vi "Configure.vi"(8 "error in (no error)":errorcluster, 11 "AOTF in":refnum<class "AOTF.lvclass">) -> (0 "error out":errorcluster, 2 "cancelled?":bool, 3 "AOTF out":refnum<class "AOTF.lvclass">)   [LabVIEW 2012, in "AOTF.lvclass"]
doc: "The configure method configures the details for the RabbitMQ connection. \n\nIn the derived class, make a call to the parent for setting these parameters."
uses:
  AOTF.lvclass
  <vilib>/Utility/miscctls.llb/LVPointTypeDef.ctl
  AOTF.lvclass/AOTF.ctl
  <vilib>/Distrio/Murmex/Murmex/Murmex.lvclass
  Controls/LUT path cluster.ctl
panel:
  in  "Tab Control":enum32{"Comport", "Debug"}(tab)
  in  "DO lines":tag
  in  "AO channel":tag
  in  "LUT561":path=path "D:/CLSM_Project/AOTF/561nm.txt" caption="LUT 561nm"
  in  "LUT515":path=path "D:/CLSM_Project/AOTF/515nm.txt" caption="LUT 515nm"
  in  "LUT491":path=path "D:/CLSM_Project/AOTF/491nm.txt" caption="LUT 491nm"
  in  "LUT445":path=path "D:/CLSM_Project/AOTF/445nm.txt" caption="LUT 445nm"
  in  "LUT405":path=path "D:/CLSM_Project/AOTF/405nm.txt" caption="LUT 405nm"
  in  "button::configure murmex":bool
  in  "button::ok":bool
  in  "button::cancel":bool
  # "RabbitMQ parameters"
  # "Window position"
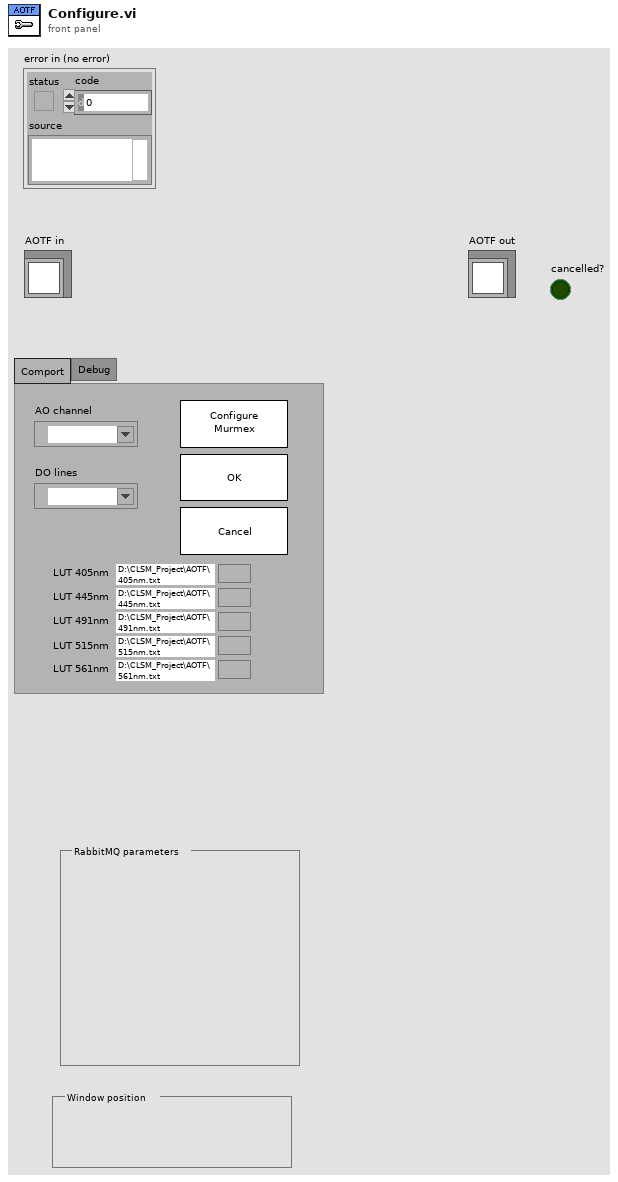
[diagram p1: front panel]
types:
  T1 = typedef "LVPointTypeDef.ctl" = cluster{"Horizontal":i16, "Vertical":i16}
  T2 = typedef "LUT path cluster.ctl" = cluster{"LUT path Array":path[]}
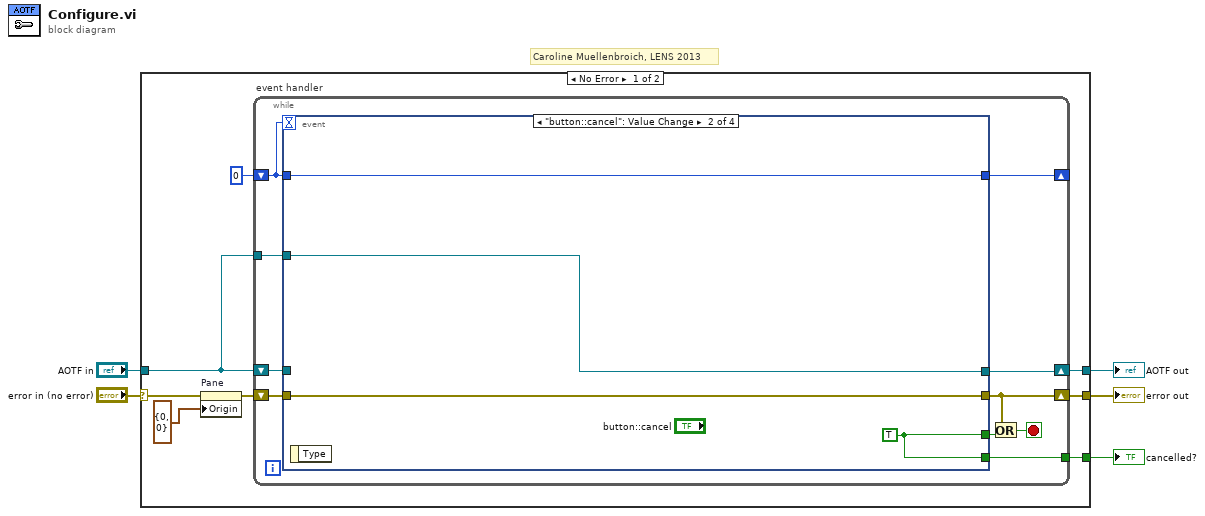
[diagram p0: block diagram]
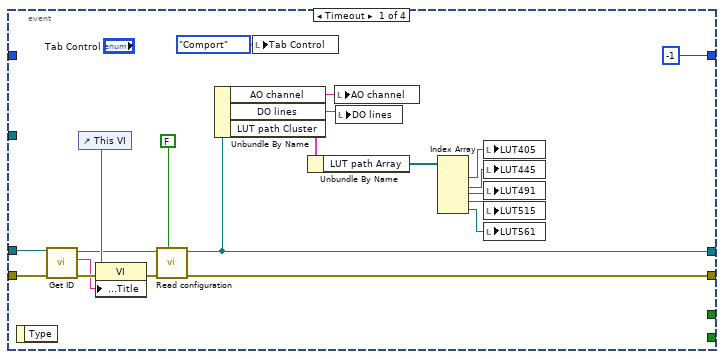
[diagram p2: hidden frame]
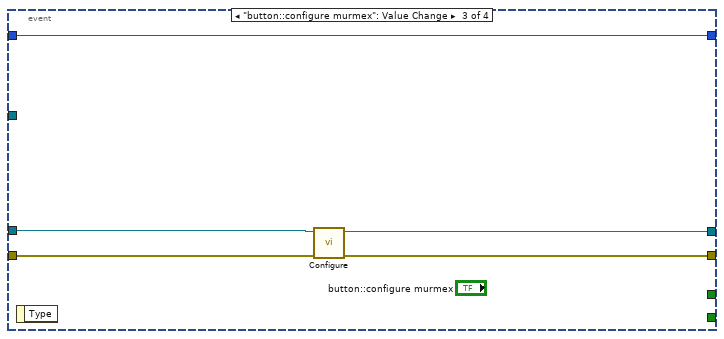
[diagram p3: hidden frame]
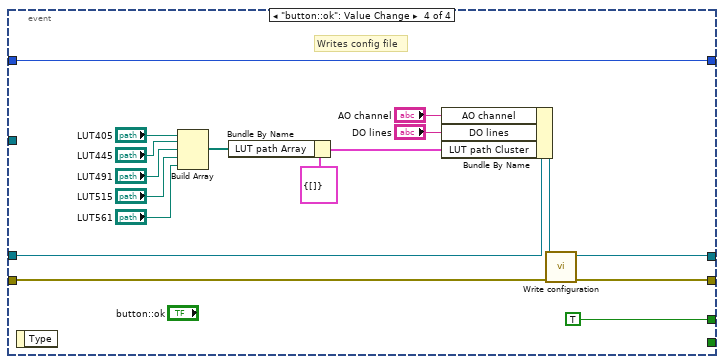
[diagram p4: hidden frame]
diagram:
  # "Caroline Muellenbroich, LENS 2013"
  n1 = case shown="No Error" "error in (no error)" {
    selector: "error in (no error)" -> [w11 w71]
    tunnel: "AOTF in" -> [w12 w72]
    tunnel: [w8 w71] -> w1
    tunnel: [w7 w72] -> w3
    tunnel: [w6 _] -> w2
    frame No Error {
      n2 = property on="Pane" class="Pane"(error in=w11, "Origin"=T1 {"Horizontal"=0, "Vertical"=0}) -> (error out=w10:errorcluster)  [unwired: 1 in, 1 out]
      n3 = while "event handler" {
        shift-right: [w23] -> _
        shift-left: 0 -> [w14]
        shift-right: [w19] -> w7
        shift-left: w12 -> [w22]
        tunnel: w12 -> [w21]
        shift-right: [w17] -> w8
        shift-left: w10 -> [w20]
        tunnel: [w15] -> w6
        stop <- w18 stop-if-true
        n4 = event shown="[1] \"button::cancel\": Value Change" {
          selector: _ -> [_ _ _ _]
          dyn-events: _ -> [_ _ _ _]
          timeout: w14 -> [_ _ _ _]
          tunnel: w14 -> [_ w48 w53 w70]
          tunnel: [-1 w48 w53 w70] -> w23
          tunnel: w22 -> [w40 _ w50 w67]
          tunnel: w21 -> [_ w45 _ _]
          tunnel: w20 -> [w43 w46 w49 w65]
          tunnel: [w35 w45 w51 w68] -> w19
          tunnel: [w34 w46 w52 w69] -> w17
          tunnel: [_ w47 _ TRUE ("force loading?")] -> w16
          tunnel: [_ w47 _ _] -> w15
          event Timeout {
            n5 = event-data() -> ()  [unwired: 1 in, 1 out]
            n6 = call <vilib>:"Get ID.vi"("error in (no error)"=w43, "Murmex in"=w40) -> ("error out"=w41:errorcluster, "component id"=w39:string, "Murmex out"=w37:refnum<class "AOTF.lvclass">)  [unwired: 7 in]
            n7 = control-ref of="This VI"() -> (w42:refnum<vi>)
            n8 = property class="VI"(reference=w42, error in=w41, "Front Panel.Title"=w39) -> (error out=w38:errorcluster)  [unwired: 1 out]
            n9 = call-dynamic "Read configuration.vi"("force loading?"=FALSE, "error in (no error)"=w38, "AOTF in"=w37) -> ("error out"=w34:errorcluster, "AOTF out"=w35:refnum<class "AOTF.lvclass">)  [unwired: 7 in]
            n10 = Unbundle By Name(w35) -> ("AO channel"=w25:tag, "DO lines"=w24:tag, "LUT path Cluster"=w32:cluster{"LUT path Array":path[]})
            n11 = local write "Tab Control"(enum32{"Comport", "Debug"}."Comport" ("Tab Control")) -> ()
            n12 = Unbundle By Name(w32) -> ("LUT path Array"=w31:path[])
            n13 = local write "AO channel"(w25) -> ()
            n14 = local write "DO lines"(w24) -> ()
            n15 = Index Array(array=w31) -> (element #1=w30:path, element #2=w29:path, element #3=w28:path, element #4=w27:path, element #5=w26:path)  [unwired: 5 in]
            n16 = local write "LUT405"(w30) -> ()
            n17 = local write "LUT445"(w29) -> ()
            n18 = local write "LUT491"(w28) -> ()
            n19 = local write "LUT515"(w27) -> ()
            n20 = local write "LUT561"(w26) -> ()
          }
          event "button::cancel": Value Change {
            w47 = TRUE ("force loading?")
            n21 = event-data() -> ()  [unwired: 1 in, 1 out]
          }
          event "button::configure murmex": Value Change {
            n22 = event-data() -> ()  [unwired: 1 in, 1 out]
            n23 = call-parent "Configure.vi"("error in (no error)"=w49, "Murmex in"=w50) -> ("error out"=w52:errorcluster, "Murmex out"=w51:refnum<class "AOTF.lvclass">)  [unwired: 7 in, 1 out]
          }
          event "button::ok": Value Change {
            # "Writes config file"
            n24 = event-data() -> ()  [unwired: 1 in, 1 out]
            n25 = Build Array("LUT405", "LUT445", "LUT491", "LUT515", "LUT561") -> (w63:path[])
            n26 = Bundle By Name(cluster=T2 {"LUT path Array"=[]} ("LUT path Cluster"), "LUT path Array"=w63) -> (w57:T2)
            n27 = Bundle By Name(cluster=w67, "AO channel"="AO channel", "DO lines"="DO lines", "LUT path Cluster"=w57) -> (w66:refnum<class "AOTF.lvclass">)
            n28 = call-dynamic "Write configuration.vi"("error in (no error)"=w65, "AOTF in"=w66) -> ("error out"=w69:errorcluster, "AOTF out"=w68:refnum<class "AOTF.lvclass">)  [unwired: 8 in]
          }
        }
        n29 = Or(x=w17, y=w16) -> (x .or. y?=w18:bool)
      }
    }
    frame Error {
    }
  }
  "error out" <- w1
  "AOTF out" <- w3
  "cancelled?" <- w2
